vi "LEBITVacuum.ParseLockedSectionsArray.vi"(1 "LockedSectionsArray":string[](array[string]), 4 "SavedLockedSectionsArray":string[][](array[string])) -> (15 "LockedSectionsArrayOut":string[](array[string]), 18 "LockedSectionsValueArray":i16[](array[numeric]))   [LabVIEW 2012, in "LEBITVacuum.lvlib"]
uses:
  LEBITVacuum.lvlib
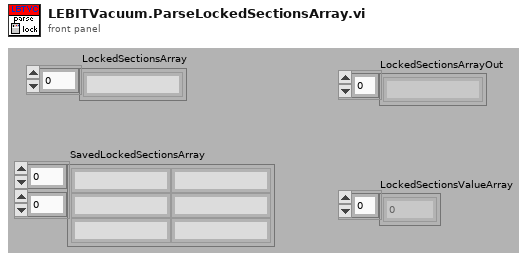
[diagram p1: front panel]
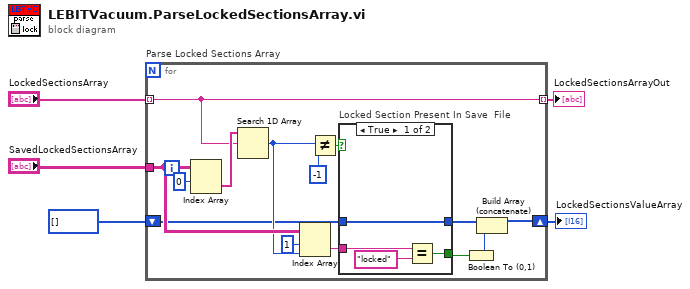
[diagram p0: block diagram]
diagram:
  n1 = for "Parse Locked Sections Array" {
    tunnel: "SavedLockedSectionsArray" -> [w13]
    tunnel: "LockedSectionsArray" -> [w17] mode=indexing
    tunnel: [w17] -> w3 mode=indexing
    shift-right: [w8] -> w1
    shift-left: i16[] [] ("LockedSectionsValueArray") -> [w10]
    n2 = Index Array(array=w13, index (row)=0 ("index")) -> (element=w18:string[])  [unwired: 1 in]
    n3 = Search 1D Array(1D array=w18, element=w17) -> (index of element=w11:i32)  [unwired: 1 in]
    n4 = Index Array(array=w13, index (row)=1, index (col)=w11) -> (element=w14:string)
    n5 = Not Equal?(x=w11, y=-1) -> (x != y?=w16:bool)
    n6 = case "Locked Section Present In Save  File" shown="True" w16 {
      tunnel: w14 -> [w23 _]
      tunnel: [w21 _] -> w7
      tunnel: w10 -> [w20 w24]
      tunnel: [w20 w24] -> w9
      frame True {
        n7 = Equal?(x=w23, y="locked") -> (x = y?=w21:bool)
      }
      frame False {
      }
    }
    n8 = Boolean To (0,1)(Boolean=w7) -> (0, 1=w6:i16)
    n9 = Build Array (concatenate)(w9, w6) -> (w8:i16[])
  }
  "LockedSectionsArrayOut" <- w3
  "LockedSectionsValueArray" <- w1
